vi "CallEngine.vi"(8 "error in (no error)":errorcluster, 10 "RT_Game.lvlib:Engine.lvclass":refnum<class "Engine.lvclass">, 11 "Pong in":refnum<class "Pong.lvclass">) -> (0 "error out":errorcluster, 2 "RT_Game.lvlib:Engine.lvclass 2":refnum<class "Engine.lvclass">, 3 "Pong out":refnum<class "Pong.lvclass">)   [LabVIEW 2019, in "RT_Game.lvlib" / "Pong.lvclass"]
uses:
  Pong.lvclass
  Engine/Engine.lvclass
  Engine/Engine.lvclass/Engine.ctl
  Engine/Write delta_t.vi
  Game/Game.lvclass
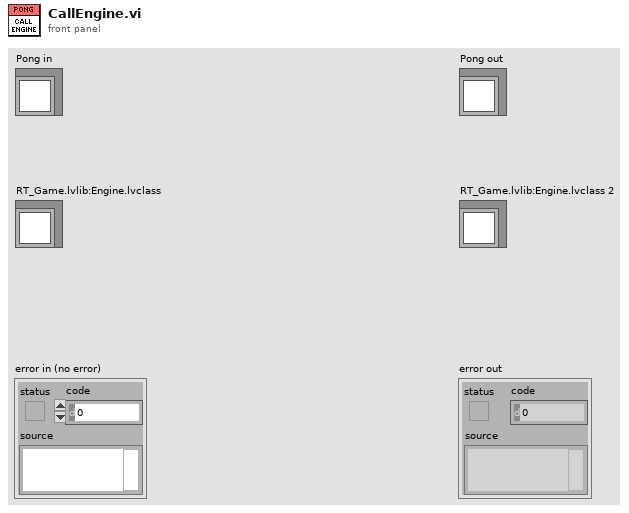
[diagram p1: front panel]
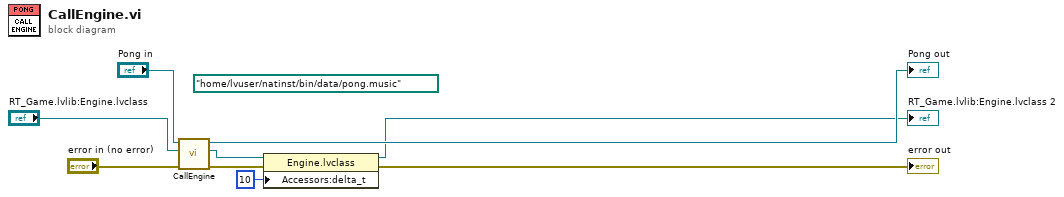
[diagram p0: block diagram]
diagram:
  (unwired) path "/home/lvuser/natinst/bin/data/pong.music" ("Path")
  n1 = call-parent "CallEngine.vi"("error in (no error)"="error in (no error)", "RT_Game.lvlib:Engine.lvclass"="RT_Game.lvlib:Engine.lvclass", "Game in"="Pong in") -> ("error out"=w9:errorcluster, "RT_Game.lvlib:Engine.lvclass 2"=w3:refnum<class "Engine.lvclass">, "Game out"=→"Pong out":refnum<class "Pong.lvclass">)  [unwired: 6 in]
  n2 = property class="Engine.lvclass"(reference=w3, error in=w9, "Accessors:delta_t"=u16 10 ("delta_t")) -> (reference out=→"RT_Game.lvlib:Engine.lvclass 2":refnum<class "Engine.lvclass">, error out=→"error out":errorcluster)
